vi "CRYUpdate Unicode MultCol Listbox Headers.vi"(6 "Caption":string, 7 "Interpret as Unicode (T)":bool=TRUE, 8 "error in (no error)":errorcluster, 9 "Row Headers[]":string[](array[string]), 10 "Column Headers[]":string[](array[string]), 11 "Multicolumn Listbox Ref":refnum<vi>) -> (0 "error out":errorcluster, 3 "Multicolumn Listbox Ref":refnum<vi>)   [LabVIEW 2013]
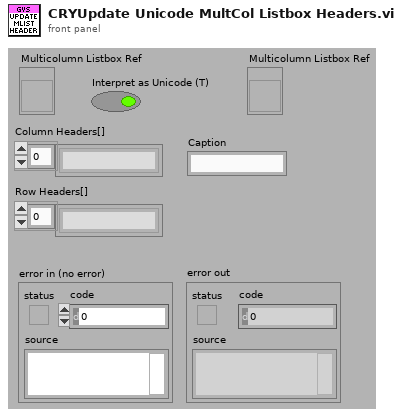
[diagram p1: front panel]
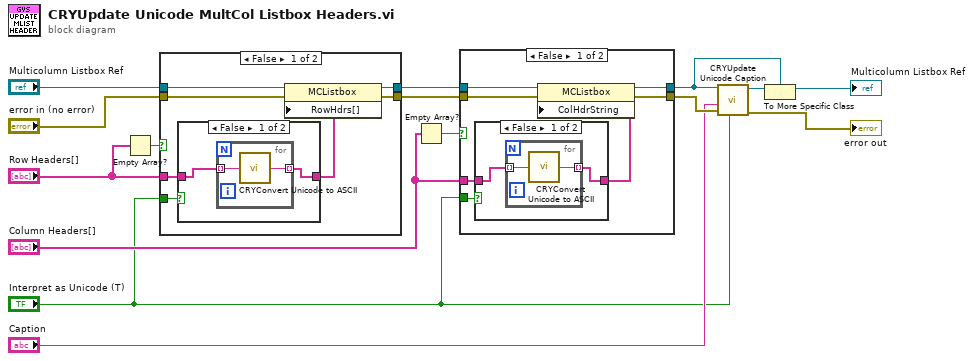
[diagram p0: block diagram]
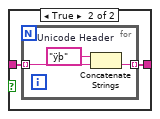
[diagram p2: hidden frame]
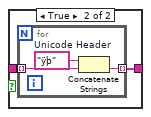
[diagram p4: hidden frame]
diagram:
  n1 = Empty Array?(array="Row Headers[]") -> (empty?=w12:bool)
  n2 = case shown="False" w12 {
    tunnel: "Row Headers[]" -> [w22 _]
    tunnel: "Multicolumn Listbox Ref" -> [w20 w33]
    tunnel: "error in (no error)" -> [w19 w32]
    tunnel: [w18 w33] -> w13
    tunnel: "Interpret as Unicode (T)" -> [w17 _]
    tunnel: [w16 w32] -> w8
    frame False {
      n3 = case shown="False" w17 {
        tunnel: w22 -> [w24 w28]
        tunnel: [w23 w27] -> w21
        frame False {
          n4 = for {
            tunnel: w24 -> [w26] mode=indexing
            tunnel: [w25] -> w23 mode=indexing
            n5 = call "CRYConvert Unicode to ASCII.vi"("Unicode"=w26) -> ("ASCII"=w25:string)  [unwired: 4 in]
          }
        }
        frame True {
          n6 = for {
            tunnel: w28 -> [w31] mode=indexing
            tunnel: [w30] -> w27 mode=indexing
            w29 = "ÿþ"  # Unicode Header
            n7 = Concatenate Strings(w29, w31) -> (w30:string)
          }
        }
      }
      n8 = property class="MCListbox"(reference=w20, error in=w19, "RowHdrs[]"=w21) -> (reference out=w18:refnum<vi>, error out=w16:errorcluster)
    }
    frame True {
    }
  }
  n9 = Empty Array?(array="Column Headers[]") -> (empty?=w9:bool)
  n10 = case shown="False" w9 {
    tunnel: "Column Headers[]" -> [w40 _]
    tunnel: [w39 w51] -> w7
    tunnel: w8 -> [w37 w51]
    tunnel: w13 -> [w36 w50]
    tunnel: "Interpret as Unicode (T)" -> [w35 _]
    tunnel: [w34 w50] -> w4
    frame False {
      n11 = case shown="False" w35 {
        tunnel: w40 -> [w42 w46]
        tunnel: [w41 w45] -> w38
        frame False {
          n12 = for {
            tunnel: w42 -> [w44] mode=indexing
            tunnel: [w43] -> w41 mode=indexing
            n13 = call "CRYConvert Unicode to ASCII.vi"("Unicode"=w44) -> ("ASCII"=w43:string)  [unwired: 4 in]
          }
        }
        frame True {
          n14 = for {
            tunnel: w46 -> [w49] mode=indexing
            tunnel: [w48] -> w45 mode=indexing
            w47 = "ÿþ"  # Unicode Header
            n15 = Concatenate Strings(w47, w49) -> (w48:string)
          }
        }
      }
      n16 = property class="MCListbox"(reference=w36, error in=w37, "ColHdrString"=w38) -> (reference out=w34:refnum<vi>, error out=w39:errorcluster)
    }
    frame True {
    }
  }
  n17 = call "CRYUpdate Unicode Caption.vi"("Interpret as Unicode (T)"="Interpret as Unicode (T)", "error in (no error)"=w7, "Caption"="Caption", "Control Reference"=w4) -> ("error out"=→"error out":errorcluster, "Control Reference"=w5:refnum<vi>)  [unwired: 4 in]
  n18 = To More Specific Class(target class=w4, reference=w5) -> (specific class reference=→"Multicolumn Listbox Ref":refnum<vi>)  [unwired: 1 in, 1 out]
